vi "TurnDegrees to MM Setpoints.vi"(2 "Turn Degrees":dbl) -> (0 "Right MM Setpoint":dbl, 1 "Left MM Setpoint":dbl)   [LabVIEW 2018]
panel:
  in  "Track Width":dbl
  # "Test text."
  # "CURRENTLY STUB VI\n\nNot anymore because of us."
  # "Will Need to create some \nnumbers for trig in constants.vi\nFor example: Trackwidth\n\n\n\n\n\n\n\n\n\n\n\n\n\n\n\n\n\nProduct of Cyril Ng and Hermela Benyam"
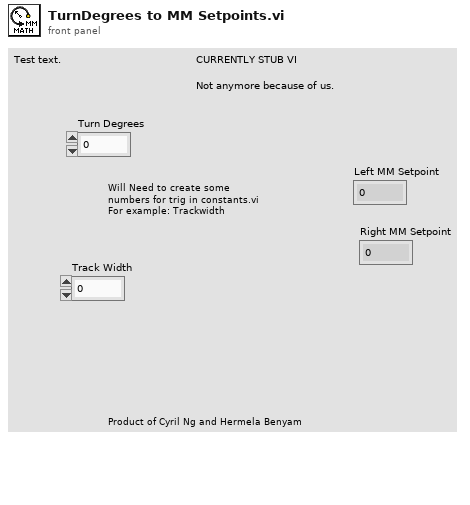
[diagram p1: front panel]
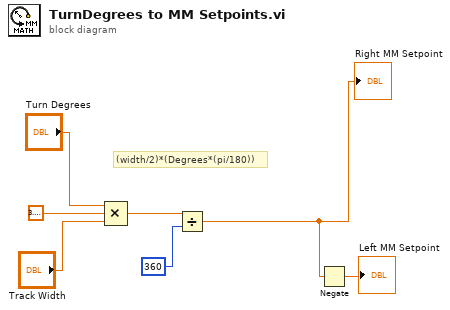
[diagram p0: block diagram]
diagram:
  # "(width/2)*(Degrees*(pi/180))"
  n1 = Compound Arithmetic op=MULTIPLY("Turn Degrees", 3.141592653589793, "Track Width") -> (w3:dbl)
  n2 = Divide(x=w3, y=360) -> (x/y=w2:dbl)
  "Right MM Setpoint" <- w2
  n3 = Negate(x=w2) -> (-x=→"Left MM Setpoint":dbl)
